vi "test.vi"() -> ()   [LabVIEW 2017]
uses:
  <vilib>/Instr/_visa.llb/VISA Configure Serial Port (Instr).vi
  <vilib>/ptbypt/NI_PtbyPt.lvlib
  <vilib>/Utility/file.llb/Write Delimited Spreadsheet (DBL).vi
panel:
  out "路径":path
  out "XY图":cluster{dbl[], dbl[]}(graph)
  out "采样频率/Hz":dbl
  out "relative seconds":dbl caption="采样周期" format="%_19f"
  out "DS力传感器值/N":dbl
  in  "DS2力传感器":refnum<visa-resource-name>="COM8"
  out "电压值/V":dbl(graph)
  in  "模拟信号串口号":refnum<visa-resource-name>="COM12"
  out "位移传感器":dbl(graph)
  in  "停止":bool
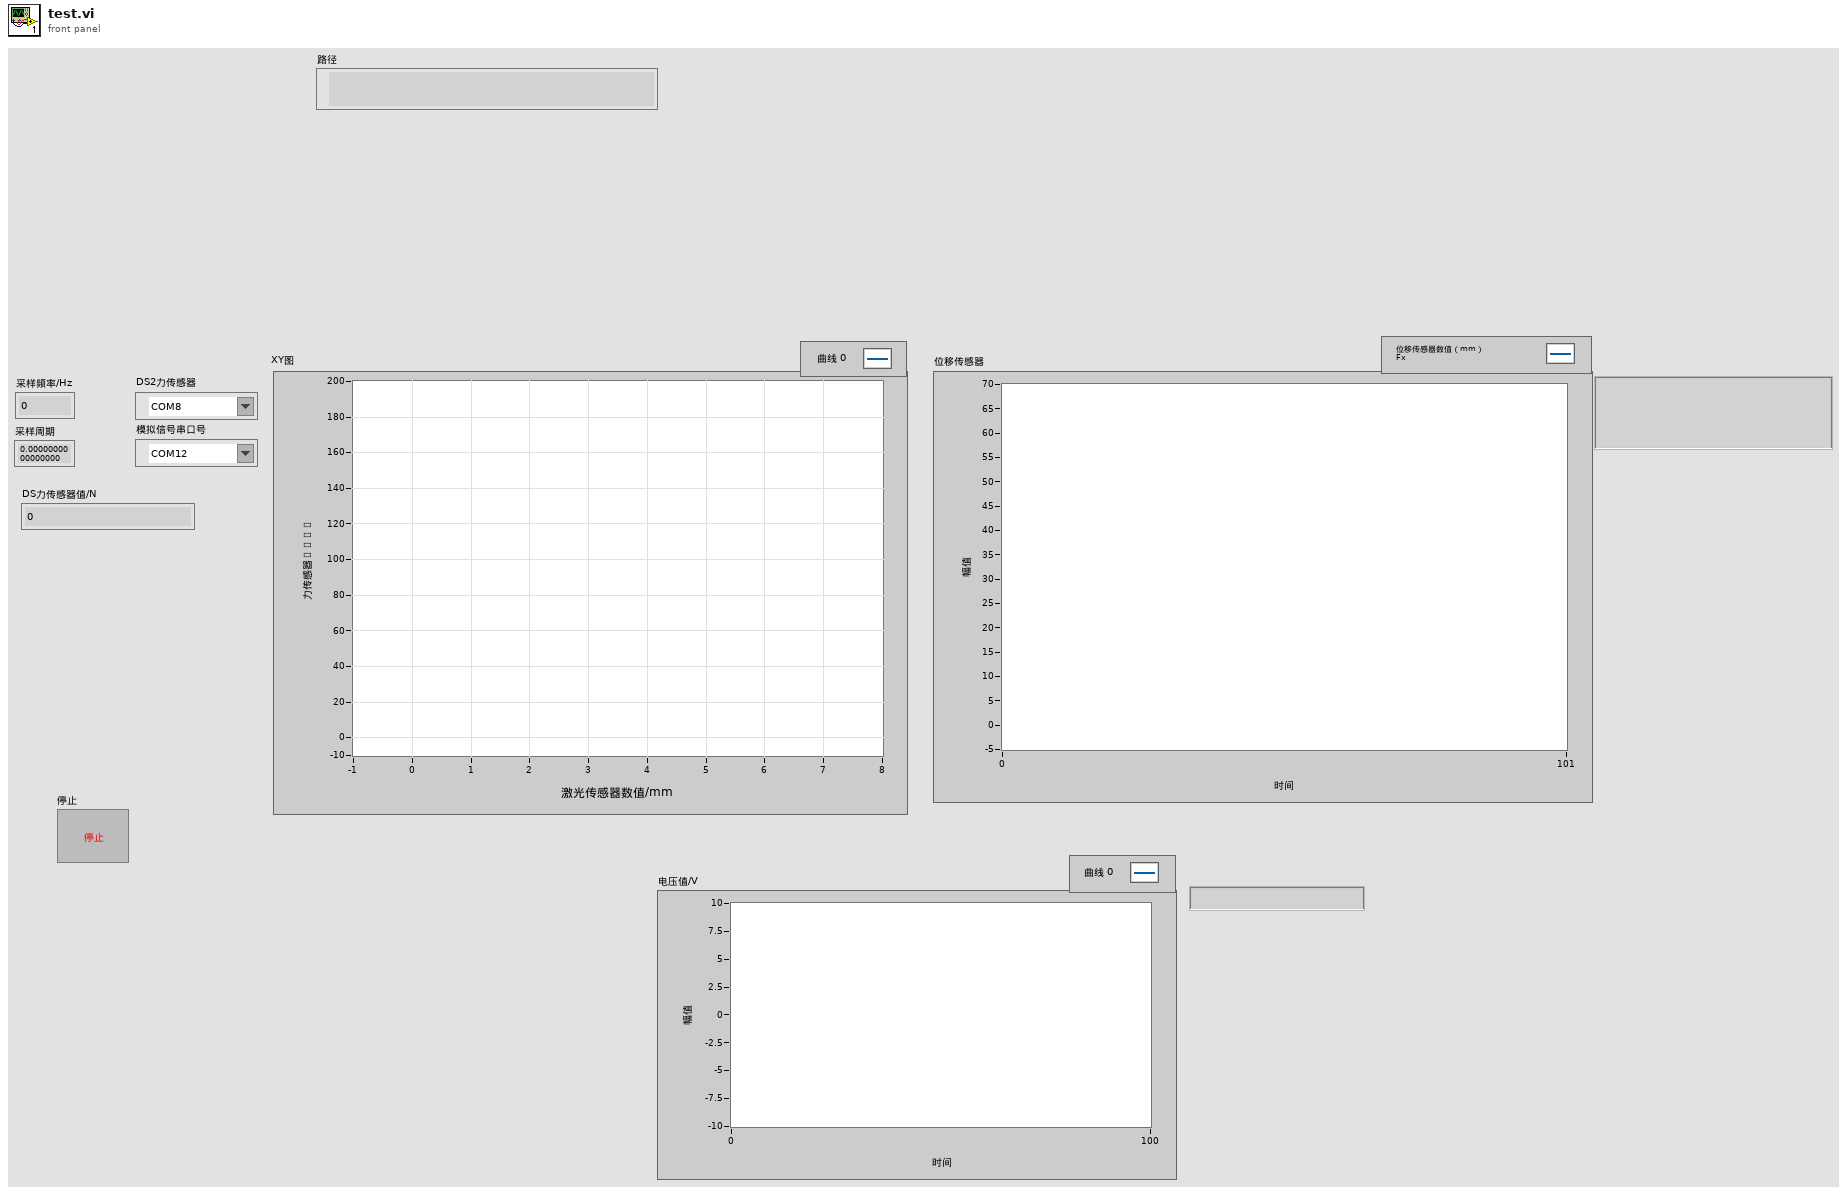
[diagram p1: front panel]
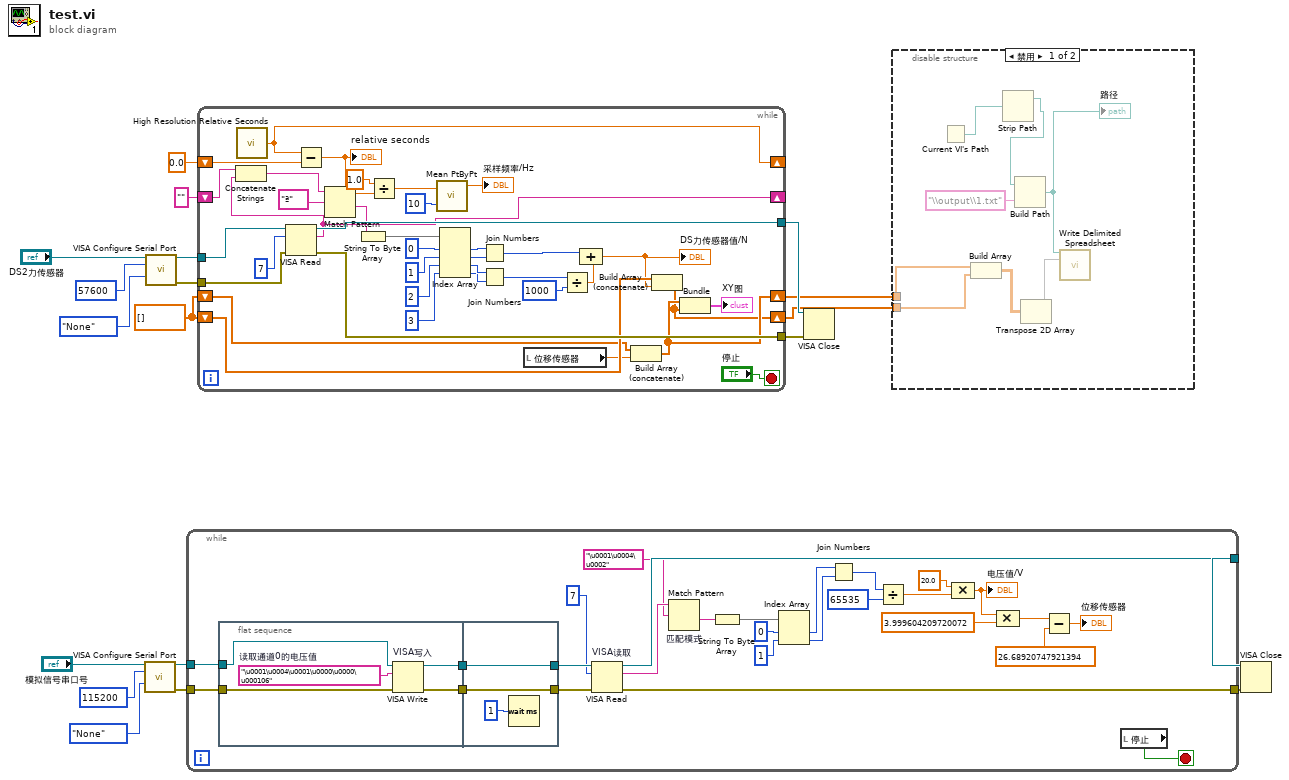
[diagram p0: block diagram]
diagram:
  w11 = dbl[] []
  n1 = call-poly "VISA Configure Serial Port"("VISA resource name"="模拟信号串口号", "baud rate (9600)"=u32 115200, "parity (0:none)"=enum16{"None", "Odd", "Even", "Mark", "Space"}."None") -> ("VISA resource name out"=w5:refnum<visa-resource-name>, "error out"=w4:errorcluster)  [unwired: 11 in]
  n2 = call-poly "VISA Configure Serial Port"("VISA resource name"="DS2力传感器", "baud rate (9600)"=u32 57600, "parity (0:none)"=enum16{"None", "Odd", "Even", "Mark", "Space"}."None") -> ("VISA resource name out"=w13:refnum<visa-resource-name>, "error out"=w14:errorcluster)  [unwired: 11 in]
  n3 = while {
    tunnel: w5 -> [w43]
    tunnel: w4 -> [w42]
    tunnel: [w41] -> w3
    tunnel: [w40] -> w2
    stop <- w37 stop-if-true
    n4 = flat-sequence {
      tunnel: w43 -> [w48]
      tunnel: w42 -> [w47]
      tunnel: [w51] -> w39
      tunnel: [w50] -> w38
      tunnel: w39 -> [w54]
      tunnel: w38 -> [w53]
      tunnel: [w54] -> w46
      tunnel: [w53] -> w45
      frame #0 {
        w49 = "\u0001\u0004\u0001\u0000\u0000\u000106"  # 读取通道0的电压值
        n5 = VISA Write "VISA写入"(VISA resource name=w48, write buffer=w49, error in (no error)=w47) -> (VISA resource name out=w50:refnum<visa-resource-name>, error out=w51:errorcluster)  [unwired: 1 out]
      }
      frame #1 {
        n6 = Wait (ms)(milliseconds to wait=u32 1 ("等待时间（毫秒）")) -> ()  [unwired: 1 out]
      }
    }
    n7 = VISA Read "VISA读取"(VISA resource name=w45, byte count=u32 7 ("字节总数"), error in (no error)=w46) -> (VISA resource name out=w41:refnum<visa-resource-name>, read buffer=w36:string, error out=w40:errorcluster)  [unwired: 1 out]
    n8 = Match Pattern "匹配模式"(string=w36, regular expression="\u0001\u0004\u0002" ("正则表达式")) -> (after substring=w32:string)  [unwired: 1 in, 3 out]
    n9 = String To Byte Array(string=w32) -> (unsigned byte array=w31:u8[])
    n10 = Index Array(array=w31, index #1=0 ("索引"), index #2=1 ("索引")) -> (element #1=w29:u8, element #2=w30:u8)
    n11 = Join Numbers(hi=w29, lo=w30) -> ((hi.lo)=w28:u16)
    n12 = Divide(x=w28, y=u16 65535) -> (x/y=w24:dbl)
    n13 = Compound Arithmetic op=MULTIPLY ("复合运算")(20.0 ("x"), w24) -> (w23:dbl)
    "电压值/V" <- w23
    n14 = Compound Arithmetic op=MULTIPLY ("复合运算")(w23, 3.999604209720072 ("值")) -> (w21:dbl)
    n15 = Subtract(x=w21, y=26.68920747921394) -> (x-y=→"位移传感器":dbl)
    n16 = local read "停止"() -> (w37:bool)
  }
  n17 = while {
    tunnel: w13 -> [w89]
    tunnel: [w92] -> w16
    tunnel: w14 -> [w90]
    tunnel: [w91] -> w15
    shift-right: [w68] -> _
    shift-left: 0.0 ("relative seconds") -> [w69]
    shift-right: [w61] -> w9
    shift-left: w11 -> [w66]
    shift-right: [w62] -> w10
    shift-left: w11 -> [w64]
    shift-right: [w59] -> _
    shift-left: "" ("read buffer") -> [w60]
    stop <- "停止" stop-if-true
    n18 = call <vilib>:"High Resolution Relative Seconds.vi"() -> ("relative seconds"=w68:dbl)
    n19 = VISA Read ("VISA读取")(VISA resource name=w89, byte count=u32 7 ("字节总数"), error in (no error)=w90) -> (VISA resource name out=w92:refnum<visa-resource-name>, read buffer=w59:string, error out=w91:errorcluster)  [unwired: 1 out]
    n20 = Concatenate Strings(w60, w59) -> (w58:string)
    n21 = Subtract(x=w68, y=w69) -> (x-y=w74:dbl)
    "relative seconds" <- w74
    n22 = Match Pattern ("匹配模式")(string=w58, regular expression="ª" ("正则表达式")) -> (after substring=w56:string)  [unwired: 1 in, 3 out]
    n23 = String To Byte Array(string=w56) -> (unsigned byte array=w85:u8[])
    n24 = Divide(x=1.0, y=w74) -> (x/y=w72:dbl)
    n25 = call <vilib>:"Mean PtByPt.vi"("x"=w72, "sample length"=10) -> ("mean"=→"采样频率/Hz":dbl)  [unwired: 2 in, 1 out]
    n26 = Index Array(array=w85, index #1=0 ("索引"), index #2=1 ("索引"), index #3=2 ("索引"), index #4=3 ("索引")) -> (element #1=w78:u8, element #2=w77:u8, element #3=w80:u8, element #4=w79:u8)
    n27 = Join Numbers(hi=w78, lo=w77) -> ((hi.lo)=w76:u16)
    n28 = Join Numbers(hi=w80, lo=w79) -> ((hi.lo)=w84:u16)
    n29 = local read "位移传感器"() -> (w65:dbl)
    n30 = Divide(x=w84, y=u16 1000) -> (x/y=w67:dbl)
    n31 = Compound Arithmetic op=ADD(w76, w67) -> (w55:dbl)
    "DS力传感器值/N" <- w55
    n32 = Build Array (concatenate)(w64, w65) -> (w62:dbl[])
    n33 = Build Array (concatenate)(w66, w55) -> (w61:dbl[])
    n34 = Bundle(w62, w61) -> (→"XY图":cluster{dbl[], dbl[]})  [unwired: 1 in]
  }
  n35 = VISA Close(VISA resource name=w16, error in (no error)=w15) -> ()  [unwired: 1 out]
  n36 = disable-structure shown="禁用" {
    disable-tunnel: w10 -> [w94 _]
    disable-tunnel: w9 -> [w93 _]
    frame Disabled {
      n37 = Current VI's Path() -> (path=w97:path)
      n38 = Build Array(w94, w93) -> (w100:dbl[][])
      n39 = Strip Path(path=w97) -> (stripped path=w96:path)  [unwired: 1 out]
      n40 = Build Path(base path=w96, name or relative path="\\output\\1.txt" ("名称或相对路径")) -> (appended path=w95:path)
      "路径" <- w95
      n41 = Transpose 2D Array(2D array=w100) -> (transposed array=w99:dbl[][])
      n42 = call-poly <vilib>:"Write Delimited Spreadsheet.vi"("file path (dialog if empty)"=w95, "2D data"=w99) -> ()  [unwired: 12 in, 2 out]
    }
    frame Enabled {
    }
  }
  n43 = VISA Close(VISA resource name=w3, error in (no error)=w2) -> ()  [unwired: 1 out]
